vi "mupExpr multiExpr multiVar example.vi"() -> ()   [LabVIEW 2015]
uses:
  mupExpr/mupExpr.lvclass/mupExpr.ctl
  mupExpr/Eval_MultiVar_MultiRes.vi
  mupExpr/SetVarVal.vi
  mupLib/mupEvalMulti.vi
  mupLib/mupSetVarValue.vi
  mupLib/mupCheckError.vi
  mupLib/mupLibPath.vi
  <vilib>/Utility/error.llb/Error Cluster From Error Code.vi
  mupExpr/mupExpr.lvclass
panel:
  out "error out":errorcluster
  out "Results":dbl[](array[numeric]) format="%#_13g"
  out "Variable Names":string[](array[string])
  in  "Expression":string="sin(w*x+c),\na*x^2+b*x+c,\na*x+b"
  in  "Variable Values":dbl[](array[numeric])=[1.0, 2.0, 3.0, 3.141592654, 1.0] format="%#_13g"
  # "This example demonstrates the evaluation of one or more multi-variable expressions.\n\n- Enter the expressions composed of any number of variables\n- Enter the value of each variable (variables are listed in alphabetical order)\n- Hit run to evaluate the expressions"
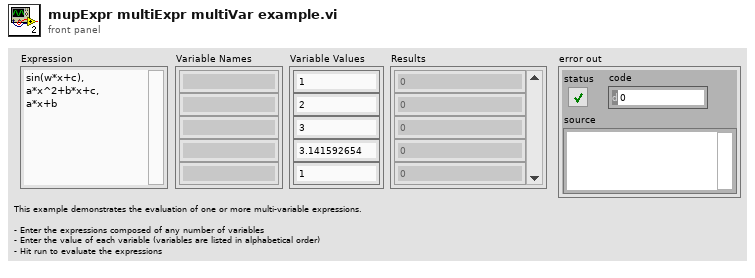
[diagram p1: front panel]
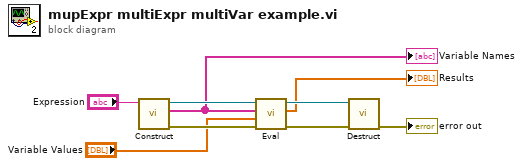
[diagram p0: block diagram]
diagram:
  n1 = call "Construct.vi"("Expression"="Expression") -> ("error out"=w7:errorcluster, "Variable Names"=w1:string[], "mupExpr out"=w6:refnum<data-value>)  [unwired: 8 in]
  "Variable Names" <- w1
  n2 = call-poly "Eval.vi"("error in (no error)"=w7, "varValues"="Variable Values", "varNames"=w1, "mupExpr in"=w6) -> ("error out"=w8:errorcluster, "Results"=→"Results":dbl[], "mupExpr out"=w9:refnum<data-value>)  [unwired: 5 in]
  n3 = call "Destruct.vi"("error in (no error)"=w8, "mupExpr in"=w9) -> ("error out"=→"error out":errorcluster)  [unwired: 9 in]
